vi "Populate Value Objects.vi"(8 "error in (no error)":errorcluster, 9 "LabVIEW types":T1[](array[typedef]), 10 "Variant":variant, 11 "Value Objects Type":refnum<class "Abs_Value.lvclass">[](array[class])) -> (0 "error out":errorcluster, 3 "Value Objects Out":refnum<class "Abs_Value.lvclass">[](array[class]))   [LabVIEW 2021, in "BT.lvlib" / "bt_WaitOn_Synch_WithValues.lvclass"]
uses:
  bt_WaitOn_Synch_WithValues.lvclass
  <vilib>/TSA/Abstract Data Classes/Abs_Types/Value/Abs_Value.lvclass
  <vilib>/Utility/Data Type/Type Definitions/Data Type.ctl
  bt_WaitOn_Synch_WithValues.lvclass/bt_WaitOn_Synch_WithValues.ctl
  <vilib>/Utility/Data Type/NI_Data Type.lvlib
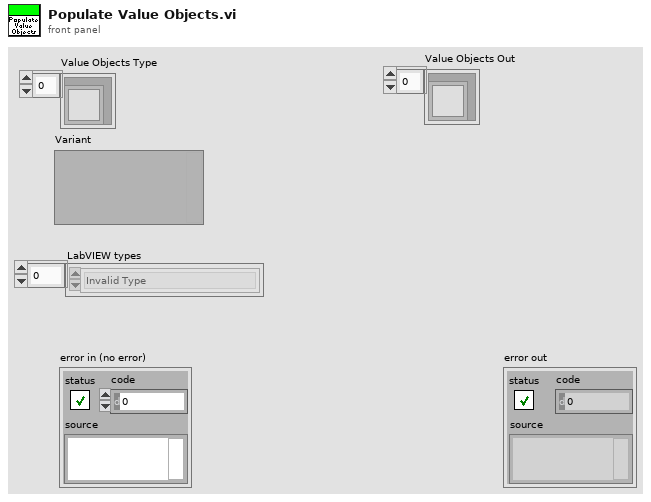
[diagram p1: front panel]
types:
  T1 = typedef "NI_Data Type.lvlib/Data Type.ctl" = enum8{"Invalid Type", "Void", "I8", "I16", "I32", "I64", "U8", "U16", "U32", "U64", "Single Float", "Double Float", "Extended Float", "Single Complex", "Double Complex", "Extended Complex", "Enum U8", "Enum U16", "Enum U32", "Enum U64", "Single Float With Unit", "Double Float With Unit", "Extended Float With Unit", "Single Complex with Unit", "Double Complex with Unit", "Extended Complex with Unit", "Boolean", "String", "Path", "Picture", "Tag", "Array", "Cluster", "Variant", "LV Variant", "Waveform", "Timestamp", "Digital Waveform", "Digital Data", "ExpressData", "Refnum", "External Data", "VI", "Poly VI", "LabVIEW Class Instance", "Fixed Point", "Set Collection", "Map Collection"}
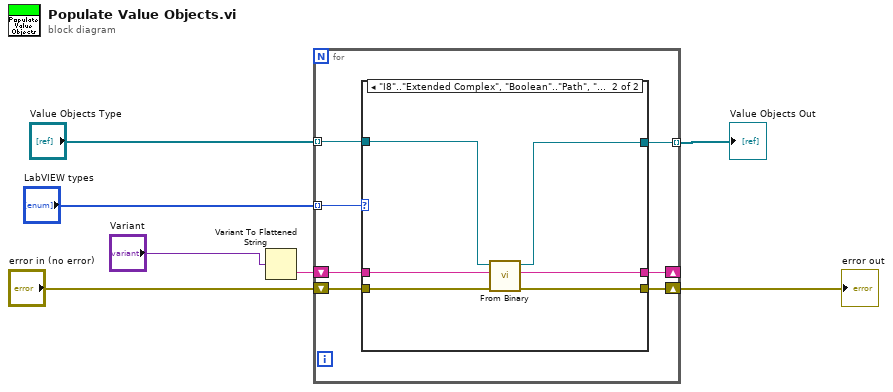
[diagram p0: block diagram]
diagram:
  n1 = Variant To Flattened String(Variant="Variant") -> (data string=w7:string)  [unwired: 1 out]
  n2 = for {
    tunnel: "Value Objects Type" -> [w14] mode=indexing
    shift-right: [w13] -> _
    shift-left: w7 -> [w12]
    tunnel: [w11] -> w1 mode=indexing
    tunnel: "LabVIEW types" -> [w8] mode=indexing
    shift-right: [w9] -> w5
    shift-left: "error in (no error)" -> [w10]
    n3 = case shown="\"I8\"..\"Extended Complex\", \"Boolean\"..\"Path\", \"Variant\"..\"Timestamp\"" w8 {
      tunnel: w14 -> [w17 w23]
      tunnel: [w16 w22] -> w13
      tunnel: w12 -> [w16 w21]
      tunnel: [w17 w20] -> w11
      tunnel: w10 -> [w15 w19]
      tunnel: [w15 w18] -> w9
      frame Default {
      }
      frame "I8".."Extended Complex", "Boolean".."Path", "Variant".."Timestamp" {
        n4 = call-dynamic "From Binary.vi"("error in (no error)"=w19, "Binary"=w21, "Type in"=w23) -> ("error out"=w18:errorcluster, "Remaining"=w22:string, "Type out"=w20:refnum<class "Abs_Value.lvclass">)  [unwired: 6 in]
      }
    }
  }
  "error out" <- w5
  "Value Objects Out" <- w1
